vi "FrequencyCoercion_2.vi"(3 "Loop Rate (Hz)":dbl=10000.0, 5 "FPGA Top-Level Clock Frequency":dbl=40000000.0) -> (0 "Actual Rate (Hz)":dbl, 2 "FPGA Ticks":u32)   [LabVIEW 2012, in "MyHostCode.lvlib"]
doc: "This VI will calculate the rate closest to the desired rate that an FPGA can produce based on the top-level clock frequency.\n\n<B>Inputs:</B>\n<B>FPGA Top-Level Clock Frequency</B> - The top-level clock rate for the FPGA.\n<B>Loop Rate (Hz)</B> - Desired rate.\n\n<B>Outputs</B>:\n<B>FPGA Ticks</B> - Number of ticks an FPGA loop should last to achieve the desired rate.\n<B>Actual Rate (Hz)</B> - Rate that will be achieved if the FPGA loop is timed to last the number of ticks specified by <B>FPGA Ticks</B>."
uses:
  MyHostCode.lvlib
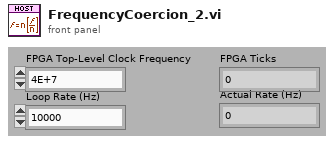
[diagram p1: front panel]
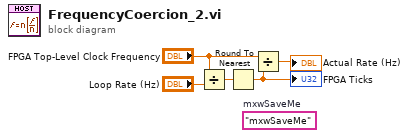
[diagram p0: block diagram]
diagram:
  (unwired) "mxwSaveMe"  # mxwSaveMe
  n1 = Divide(x="FPGA Top-Level Clock Frequency", y="Loop Rate (Hz)") -> (x/y=w2:dbl)
  n2 = Round To Nearest(number=w2) -> (nearest integer value=w1:dbl)
  "FPGA Ticks" <- w1
  n3 = Divide(x="FPGA Top-Level Clock Frequency", y=w1) -> (x/y=→"Actual Rate (Hz)":dbl)
